vi "test-DiffDrvPoseEst2-testFollowTrajectory.vi"(0 "chassisSpeedsGenerator":refnum<vi>, 1 "TRAJECTORY":T10 {"States"."POSE"."ROTATION"."SIN" format="%13.4f"; "States"."POSE"."ROTATION"."COS" format="%13.4f"; "States"."POSE"."ROTATION"."VALUE" format="%13.4f"; "States"."POSE"."TRANSLATION"."Y" format="%14.3f"; "States"."POSE"."TRANSLATION"."X" format="%14.3f"; "TotalTImeSecs" format="%20.3f"}, 2 "DiffDrivePoseEstimate":T5 {"Diff_Drive_Odom_2"."M_PrevAngle"."SIN" format="%13.4f"; "Diff_Drive_Odom_2"."M_PrevAngle"."COS" format="%13.4f"; "Diff_Drive_Odom_2"."M_PrevAngle"."VALUE" format="%13.4f"; "Diff_Drive_Odom_2"."M_GyroOffset"."SIN" format="%13.4f"; "Diff_Drive_Odom_2"."M_GyroOffset"."COS" format="%13.4f"; "Diff_Drive_Odom_2"."M_GyroOffset"."VALUE" format="%13.4f"; "Diff_Drive_Odom_2"."M_POSE_Meters"."ROTATION"."SIN" format="%13.4f"; "Diff_Drive_Odom_2"."M_POSE_Meters"."ROTATION"."COS" format="%13.4f"; "Diff_Drive_Odom_2"."M_POSE_Meters"."ROTATION"."VALUE" format="%13.4f"; "Diff_Drive_Odom_2"."M_POSE_Meters"."TRANSLATION"."Y" format="%14.3f"; "Diff_Drive_Odom_2"."M_POSE_Meters"."TRANSLATION"."X" format="%14.3f"; "Diff_Drive_Kinematics"."TrackWidth_Meters" format="%20.4f"}, 3 "DIFF_DRIVE_KINEMATICS":T8 {"TrackWidth_Meters" format="%20.4f"}, 5 "genVisionMeasurement":refnum<vi>, 7 "StartingPose":T2={"TRANSLATION"={"X"=0.0, "Y"=0.0}, "ROTATION"={"VALUE"=0.0, "COS"=1.0, "SIN"=0.0}} {"ROTATION"."SIN" format="%13.4f"; "ROTATION"."COS" format="%13.4f"; "ROTATION"."VALUE" format="%13.4f"; "TRANSLATION"."Y" format="%14.3f"; "TRANSLATION"."X" format="%14.3f"}, 9 "EndingPose":T2={"TRANSLATION"={"X"=0.0, "Y"=0.0}, "ROTATION"={"VALUE"=0.0, "COS"=1.0, "SIN"=0.0}} {"ROTATION"."SIN" format="%13.4f"; "ROTATION"."COS" format="%13.4f"; "ROTATION"."VALUE" format="%13.4f"; "TRANSLATION"."Y" format="%14.3f"; "TRANSLATION"."X" format="%14.3f"}, 11 "dt_Seconds":dbl, 12 "VisionUpdateRate":dbl, 13 "VisionUpdateDelay":dbl, 14 "CheckError":bool) -> (4 "Test Passed":bool, 6 "Output Data":T1, 15 "DataForGraph":cluster{dbl[], dbl[]}[](array[cluster]))   [LabVIEW 2019]
uses:
  <vilib>/Rock Robotics/WPI/ThirdParty/JAS_Junk/TrajLib/TypeDef/TRAJECTORY.ctl
  <vilib>/Rock Robotics/WPI/ThirdParty/JAS_Junk/TrajLib/TypeDef/TRAJ_STATE.ctl
  <vilib>/Rock Robotics/WPI/ThirdParty/JAS_Junk/TrajLib/TypeDef/POSE2D.ctl
  <vilib>/Rock Robotics/WPI/ThirdParty/JAS_Junk/TrajLib/TypeDef/TRANSLATION2D.ctl
  <vilib>/Rock Robotics/WPI/ThirdParty/JAS_Junk/TrajLib/TypeDef/ROTATION2D.ctl
  <vilib>/Rock Robotics/WPI/ThirdParty/JAS_Junk/TrajLib/TypeDef/DIFF_DRIVE_KINEMATICS.ctl
  <vilib>/Rock Robotics/WPI/ThirdParty/JAS_Junk/TrajLib/TypeDef/DIFF_DRIVE_POSE_EST2.ctl
  <vilib>/Analysis/Matrix/Datatypes/RealMatrix.ctl
  <vilib>/Rock Robotics/WPI/ThirdParty/JAS_Junk/TrajLib/TypeDef/TIME_INTERPOLATABLE_VARIANT.ctl
  <vilib>/Rock Robotics/WPI/ThirdParty/JAS_Junk/TrajLib/TypeDef/DIFF_DRIVE_ODOM2.ctl
  <vilib>/Rock Robotics/WPI/ThirdParty/JAS_Junk/TrajLib/Conv_Deg_Radians.vi
  <vilib>/Rock Robotics/WPI/ThirdParty/JAS_Junk/TrajLib/VI/Util_GetTime_U32.vi
  <vilib>/Rock Robotics/WPI/ThirdParty/JAS_Junk/TrajLib/Pose2d_TransformBy.vi
  <vilib>/Rock Robotics/WPI/ThirdParty/JAS_Junk/TrajLib/VI/TimeInterpPose2d_CleanUp.vi
  <vilib>/Rock Robotics/WPI/ThirdParty/JAS_Junk/TrajLib/Rotation2d_RotateBy.vi
  <vilib>/Rock Robotics/WPI/ThirdParty/JAS_Junk/TrajLib/Rotation2d_UnaryMinus.vi
  <vilib>/Rock Robotics/WPI/ThirdParty/JAS_Junk/TrajLib/Util_CalcDist.vi
  <vilib>/Rock Robotics/WPI/ThirdParty/JAS_Junk/TrajLib/Translation2d_RotateBy.vi
  <vilib>/Rock Robotics/WPI/ThirdParty/JAS_Junk/TrajLib/Translation2d_Plus.vi
  <vilib>/Rock Robotics/WPI/ThirdParty/JAS_Junk/TrajLib/Pose2d_New_TRRO.vi
  <vilib>/Rock Robotics/WPI/ThirdParty/JAS_Junk/TrajLib/Rotation2d_CreateXY.vi
  <vilib>/Rock Robotics/WPI/ThirdParty/JAS_Junk/TrajLib/VI/Util_GetTime_U64.vi
  <vilib>/gmath/interp.llb/Search Ordered Table.vi
  <vilib>/Rock Robotics/WPI/ThirdParty/JAS_Junk/TrajLib/Trajectory_Library.lvlib
  <vilib>/Analysis/Matrix/NI_Matrix.lvlib
panel:
  in  "UseVIsion":bool=TRUE
  out "error out":errorcluster
  in  "error in (no error)":errorcluster
  # "<3, 1>"
  # "<3, 3>"
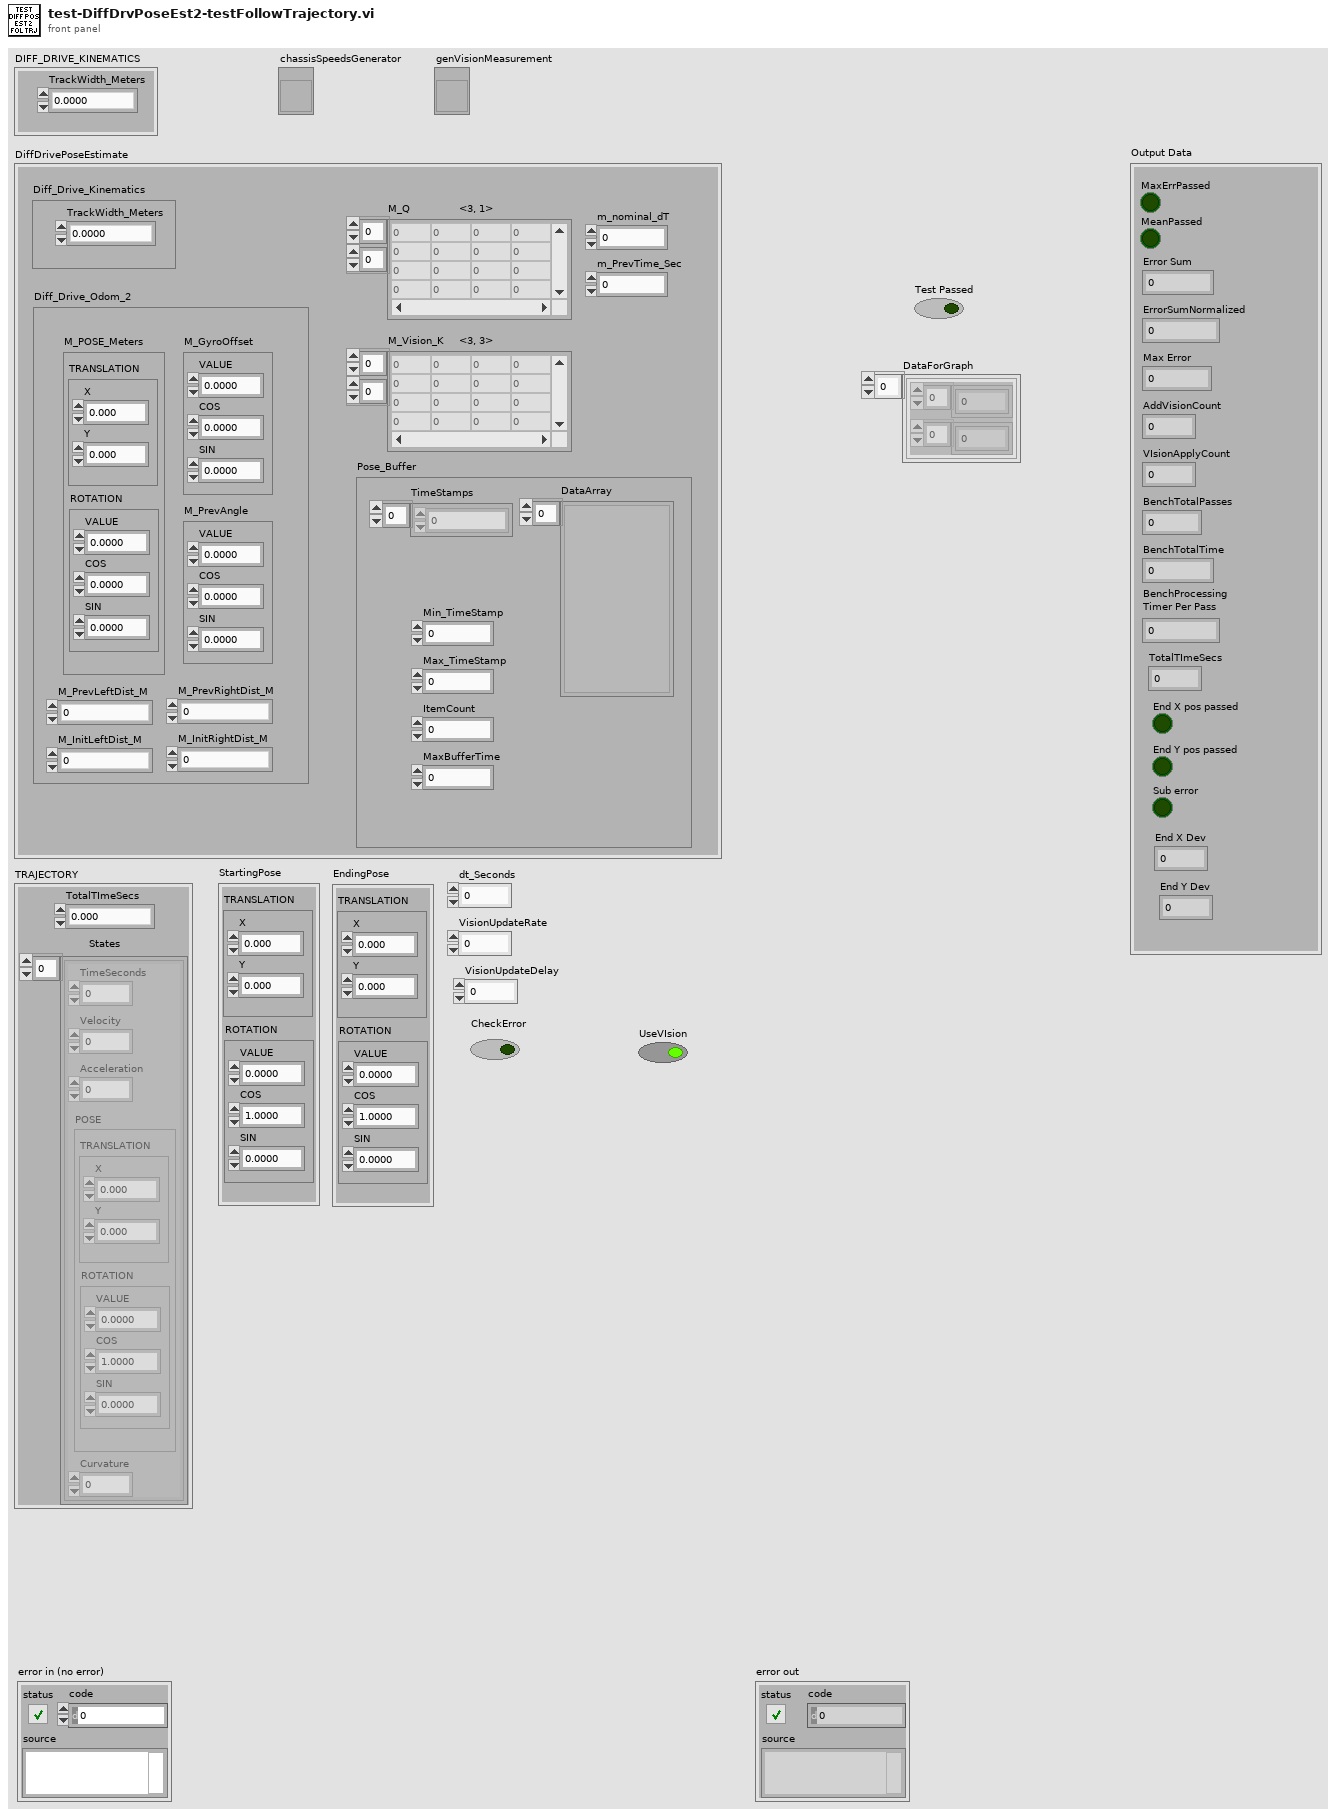
[diagram p1: front panel]
types:
  T1 = cluster{"MaxErrPassed":bool, "MeanPassed":bool, "Error Sum":dbl, "ErrorSumNormalized":dbl, "Max Error":dbl, "AddVisionCount":i32, "VIsionApplyCount":i32, "BenchTotalPasses":dbl, "BenchTotalTime":dbl, "BenchProcessing \nTimer Per Pass":dbl, "TotalTImeSecs":dbl, "End X pos passed":bool, "End Y pos passed":bool, "Sub error":bool, "End X Dev":dbl, "End Y Dev":dbl}
  T2 = typedef "Trajectory_Library.lvlib/POSE2D.ctl" = cluster{"TRANSLATION":T3, "ROTATION":T4}
  T3 = typedef "Trajectory_Library.lvlib/TRANSLATION2D.ctl" = cluster{"X":dbl, "Y":dbl}
  T4 = typedef "Trajectory_Library.lvlib/ROTATION2D.ctl" = cluster{"VALUE":dbl, "COS":dbl, "SIN":dbl}
  T5 = typedef "Trajectory_Library.lvlib/DIFF_DRIVE_POSE_EST2.ctl" = cluster{"M_Vision_K":T6, "m_nominal_dT":dbl, "m_PrevTime_Sec":dbl, "Pose_Buffer":T7, "Diff_Drive_Kinematics":T8, "Diff_Drive_Odom_2":T9, "M_Q":T6}
  T6 = typedef "NI_Matrix.lvlib/RealMatrix.ctl" = dbl[][]
  T7 = typedef "Trajectory_Library.lvlib/TIME_INTERPOLATABLE_VARIANT.ctl" = cluster{"TimeStamps":dbl[], "DataArray":variant[], "Min_TimeStamp":dbl, "Max_TimeStamp":dbl, "ItemCount":i32, "MaxBufferTime":dbl}
  T8 = typedef "Trajectory_Library.lvlib/DIFF_DRIVE_KINEMATICS.ctl" = cluster{"TrackWidth_Meters":dbl}
  T9 = typedef "Trajectory_Library.lvlib/DIFF_DRIVE_ODOM2.ctl" = cluster{"M_POSE_Meters":T2, "M_GyroOffset":T4, "M_PrevAngle":T4, "M_PrevLeftDist_M":dbl, "M_PrevRightDist_M":dbl, "M_InitLeftDist_M":dbl, "M_InitRightDist_M":dbl}
  T10 = typedef "Trajectory_Library.lvlib/TRAJECTORY.ctl" = cluster{"TotalTImeSecs":dbl, "States":T11[]}
  T11 = typedef "Trajectory_Library.lvlib/TRAJ_STATE.ctl" = cluster{"TimeSeconds":dbl, "Velocity":dbl, "Acceleration":dbl, "POSE":T2, "Curvature":dbl}
  T12 = typedef "Trajectory_Library.lvlib/TIME_INTERPOLATABLE_POSE2D.ctl" = cluster{"TimeStamps":dbl[], "Pose":T2[], "Min_TimeStamp":dbl, "Max_TimeStamp":dbl, "ItemCount":i32, "MaxBufferTime":dbl}
  T13 = typedef "Trajectory_Library.lvlib/TRANSFORM2D.ctl" = cluster{"TRANSLATION":T3, "ROTATION":T4, "xF":bool}
  T14 = typedef "Trajectory_Library.lvlib/CHASSIS_SPEEDS.ctl" = cluster{"vX":dbl, "vY":dbl, "vOmega":dbl}
  T15 = cluster{bool, bool, "Error Sum":dbl, dbl, dbl, i32, i32, "TotalPasses":dbl, "TotalTime":dbl, dbl, "TotalTImeSecs":dbl, bool, bool, bool, dbl, dbl}
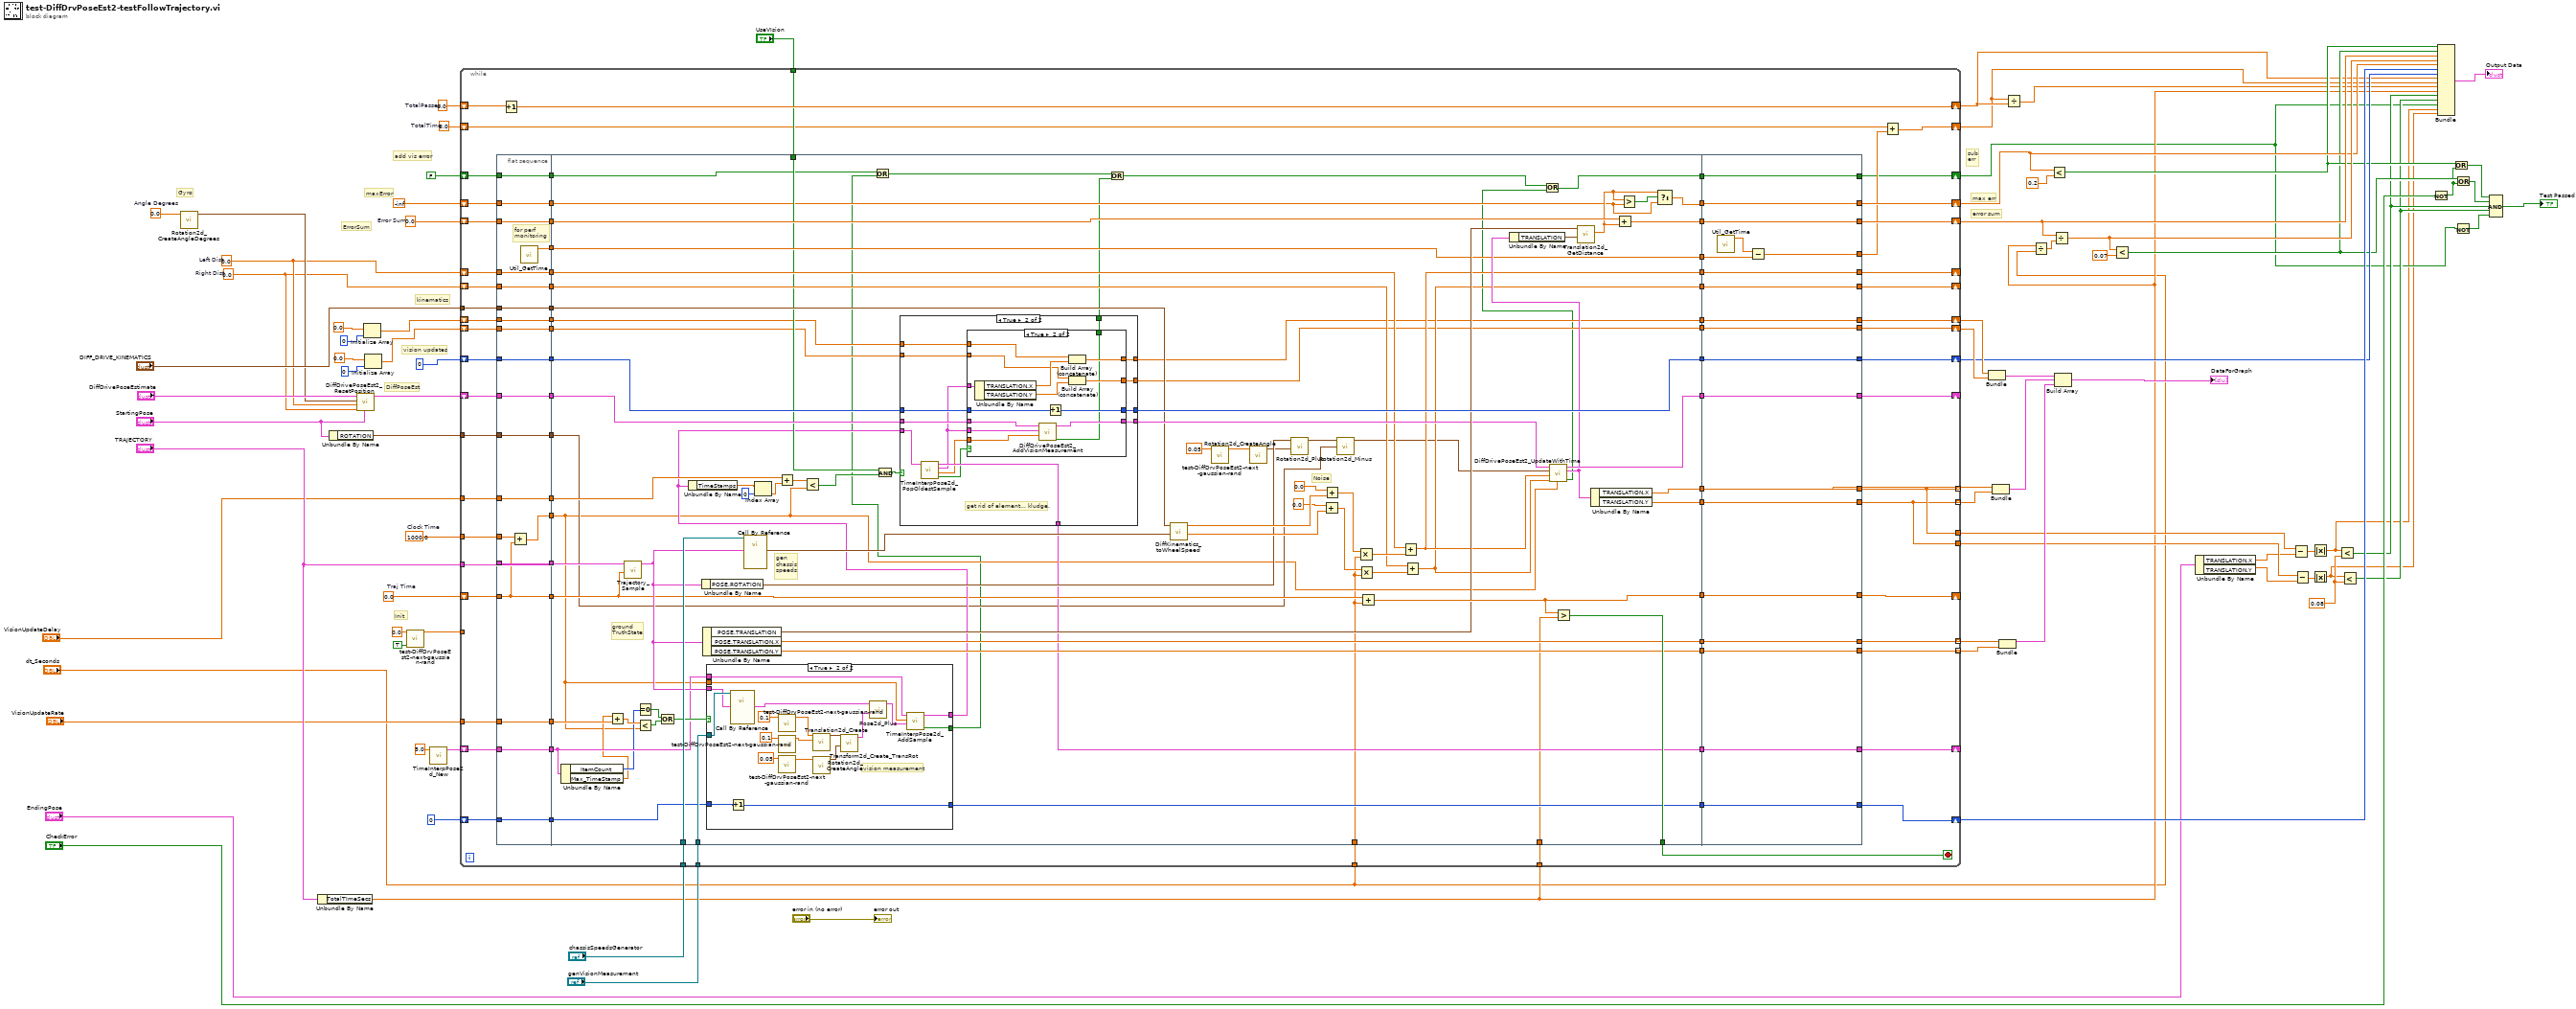
[diagram p0: block diagram]
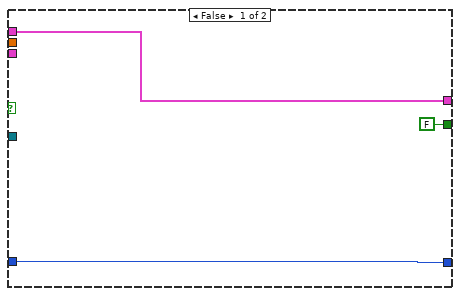
[diagram p2: hidden frame]
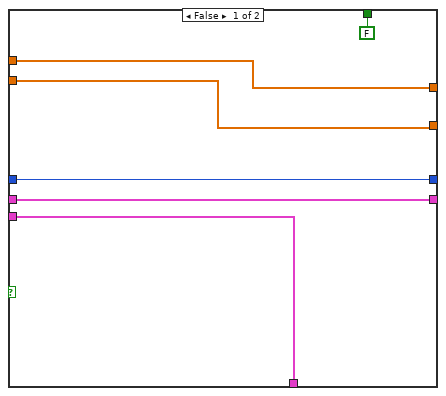
[diagram p3: hidden frame]
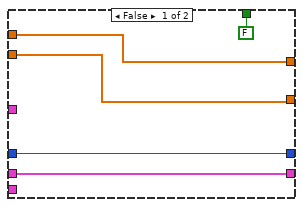
[diagram p4: hidden frame]
diagram:
  w22 = 0.08
  w47 = 1000.0  # Clock Time
  w57 = 0.0  # Angle Degrees
  w54 = 0.0  # Right Dist
  w55 = 0.0  # Left Dist
  w77 = 0.0  # TotalPasses
  w76 = 0.0  # TotalTime
  w71 = 0.0  # Error Sum
  w61 = 0.0  # Traj Time
  # "Init"
  # "sub\nerr"
  # "add vis error"
  # "max err"
  # "error sum"
  # "Gyro"
  # "ErrorSum"
  # "maxError"
  # "vision updates"
  # "kinematics"
  # "DiffPoseEst"
  n1 = call <vilib>:"Rotation2d_CreateAngleDegrees.vi"("Angle_Degrees"=w57) -> ("ROTATION"=w56:T4)  [unwired: 10 in]
  n2 = Unbundle By Name("TRAJECTORY") -> ("TotalTImeSecs"=w12:dbl)
  n3 = Unbundle By Name("StartingPose") -> ("ROTATION"=w30:T4)
  n4 = call <vilib>:"DiffDrivePoseEst2_ResetPosition.vi"("Pose"="StartingPose", "RightDistance_M"=w54, "LeftDistance_M"=w55, "Gyro"=w56, "in DiffDrivePoseEst2"="DiffDrivePoseEstimate") -> ("Out DiffDrivePoseEst2"=w58:T5)  [unwired: 6 in]
  n5 = Initialize Array(0.0, 0 ("dimension size")) -> (w42:dbl[])
  n6 = Initialize Array(0.0, 0 ("dimension size")) -> (w41:dbl[])
  n7 = call "test-DiffDrvPoseEst2-next-gaussian-rand.vi"("Init"=TRUE, "Multiplier"=0.0 ("R2")) -> ("Gaussian white noise"=w1:dbl)  [unwired: 9 in]
  n8 = call <vilib>:"TimeInterpPose2d_New.vi"("MaxTime"=5.0) -> ("TimeInterpPose"=w51:T12)  [unwired: 10 in]
  n9 = while {
    shift-right: [w162] -> _
    shift-left: w61 -> [w157]
    tunnel: "TRAJECTORY" -> [w160]
    tunnel: w12 -> [w161]
    tunnel: "VisionUpdateRate" -> [w110]
    shift-right: [w125] -> _
    shift-left: w58 -> [w159]
    tunnel: [w92] -> w62 mode=indexing
    tunnel: [w91] -> w63 mode=indexing
    shift-right: [w155] -> w32
    shift-left: 0 -> [w156]
    tunnel: [w154] -> w67 mode=indexing
    tunnel: [w153] -> w68 mode=indexing
    shift-right: [w150] -> w35
    shift-left: -inf -> [w149]
    shift-right: [w151] -> w37
    shift-left: w71 -> [w152]
    shift-right: [w87] -> w14
    shift-left: w76 -> [w88]
    shift-right: [w127] -> w15
    shift-left: w77 -> [w128]
    tunnel: "UseVIsion" -> [w126]
    shift-right: [w120] -> _
    shift-left: w55 -> [w123]
    shift-right: [w118] -> _
    shift-left: w54 -> [w121]
    tunnel: "DIFF_DRIVE_KINEMATICS" -> [w158]
    shift-right: [w113] -> _
    shift-left: w51 -> [w115]
    tunnel: "chassisSpeedsGenerator" -> [w116]
    tunnel: "genVisionMeasurement" -> [w111]
    tunnel: "VisionUpdateDelay" -> [w109]
    tunnel: w47 -> [w107]
    shift-right: [w102] -> w40
    shift-left: w42 -> [w105]
    shift-right: [w100] -> w39
    shift-left: w41 -> [w103]
    shift-right: [w96] -> w33
    shift-left: 0 -> [w97]
    tunnel: w30 -> [w93]
    tunnel: [w92] -> w28
    tunnel: [w91] -> w27
    shift-right: [w84] -> w7
    shift-left: FALSE -> [w85]
    tunnel: "dt_Seconds" -> [w82]
    tunnel: w1 -> [_]
    stop <- w148 stop-if-true
    n10 = flat-sequence {
      tunnel: w149 -> [w176]
      tunnel: w152 -> [w177]
      tunnel: w156 -> [w178]
      tunnel: w157 -> [w169]
      tunnel: w158 -> [w179]
      tunnel: w159 -> [w180]
      tunnel: w110 -> [w181]
      tunnel: w160 -> [w182]
      tunnel: [w182] -> w147
      tunnel: [w181] -> w146
      tunnel: [w180] -> w145
      tunnel: [w179] -> w144
      tunnel: [w169] -> w143
      tunnel: [w178] -> w142
      tunnel: [w177] -> w141
      tunnel: [w176] -> w140
      tunnel: [w171] -> w130
      tunnel: [w175] -> w124
      tunnel: w123 -> [w175]
      tunnel: [w174] -> w122
      tunnel: w121 -> [w174]
      tunnel: w115 -> [w173]
      tunnel: [w173] -> w114
      tunnel: w109 -> [w172]
      tunnel: [w172] -> w108
      tunnel: w107 -> [w170]
      tunnel: [w168] -> w106
      tunnel: w105 -> [w168]
      tunnel: [w167] -> w104
      tunnel: w103 -> [w167]
      tunnel: [w166] -> w98
      tunnel: w97 -> [w166]
      tunnel: [w165] -> w94
      tunnel: w93 -> [w165]
      tunnel: [w164] -> w90
      tunnel: [w163] -> w86
      tunnel: w85 -> [w163]
      tunnel: [w263] -> w148
      tunnel: w161 -> [w192]
      tunnel: w147 -> [w261]
      tunnel: w146 -> [w221]
      tunnel: w145 -> [w260]
      tunnel: w144 -> [w242]
      tunnel: w143 -> [w207]
      tunnel: w142 -> [w256]
      tunnel: w141 -> [w249]
      tunnel: w140 -> [w191]
      tunnel: [w262] -> w139
      tunnel: [w259] -> w138
      tunnel: [w258] -> w137
      tunnel: [w257] -> w136
      tunnel: [w255] -> w135
      tunnel: [w254] -> w134
      tunnel: [w253] -> w133
      tunnel: [w248] -> w132
      tunnel: [w245] -> w131
      tunnel: w130 -> [w244]
      tunnel: [w244] -> w129
      tunnel: w126 -> [w215]
      tunnel: w124 -> [w235]
      tunnel: w122 -> [w234]
      tunnel: [w231] -> w119
      tunnel: [w230] -> w117
      tunnel: w116 -> [w228]
      tunnel: w114 -> [w219]
      tunnel: [w206] -> w112
      tunnel: w111 -> [w226]
      tunnel: w108 -> [w212]
      tunnel: w106 -> [w205]
      tunnel: w104 -> [w204]
      tunnel: [w203] -> w101
      tunnel: [w202] -> w99
      tunnel: w98 -> [w201]
      tunnel: [w200] -> w95
      tunnel: w94 -> [w194]
      tunnel: w90 -> [w193]
      tunnel: w86 -> [w186]
      tunnel: [w188] -> w83
      tunnel: w82 -> [w183]
      tunnel: [w335] -> w150
      tunnel: [w336] -> w151
      tunnel: [w337] -> w153
      tunnel: [w338] -> w154
      tunnel: [w339] -> w155
      tunnel: [w340] -> w91
      tunnel: [w341] -> w92
      tunnel: [w342] -> w125
      tunnel: [w343] -> w162
      tunnel: w139 -> [w343]
      tunnel: w138 -> [w342]
      tunnel: w137 -> [w341]
      tunnel: w136 -> [w340]
      tunnel: w135 -> [w339]
      tunnel: w134 -> [w338]
      tunnel: w133 -> [w337]
      tunnel: w132 -> [w336]
      tunnel: w131 -> [w335]
      tunnel: w129 -> [w333]
      tunnel: [w332] -> w120
      tunnel: w119 -> [w332]
      tunnel: [w331] -> w118
      tunnel: w117 -> [w331]
      tunnel: [w330] -> w113
      tunnel: w112 -> [w330]
      tunnel: [w329] -> w102
      tunnel: w101 -> [w329]
      tunnel: [w328] -> w100
      tunnel: w99 -> [w328]
      tunnel: [w327] -> w96
      tunnel: w95 -> [w327]
      tunnel: [w326] -> w89
      tunnel: [w325] -> w84
      tunnel: w83 -> [w325]
      frame #0 {
        # "for perf\nmonitoring"
        n11 = Add(x=w170, y=w169) -> (x+y=w164:dbl)
        n12 = call <vilib>:"Util_GetTime.vi"() -> ("FPGA_Time_Seconds"=w171:dbl)  [unwired: 9 in, 2 out]
      }
      frame #1 {
        # "Noise"
        # "gen\nchassis\nspeeds"
        # "ground\nTruthState"
        n13 = Unbundle By Name(w219) -> ("ItemCount"=w218:i32, "Max_TimeStamp"=w217:dbl)
        n14 = Add(x=w217, y=w221) -> (x+y=w220:dbl)
        n15 = call <vilib>:"Trajectory_Sample.vi"("Time"=w207, "InputTRAJECTORY"=w261) -> ("OutputTRAJ_STATE"=w225:T11)  [unwired: 9 in]
        n16 = Equal To 0?(x=w218) -> (x = 0?=w224:bool)
        n17 = Less?(x=w220, y=w193) -> (x < y?=w223:bool)
        n18 = Compound Arithmetic op=OR(w224, w223) -> (w222:bool)
        n19 = Unbundle By Name(w225) -> ("POSE.ROTATION"=w233:T4)
        n20 = Unbundle By Name(w225) -> ("POSE.TRANSLATION"=w252:T3, "POSE.TRANSLATION.X"=w253:dbl, "POSE.TRANSLATION.Y"=w254:dbl)
        n21 = case shown="True" w222 {
          tunnel: w226 -> [_ w285]
          tunnel: w225 -> [_ w284]
          tunnel: w219 -> [w266 w273]
          tunnel: w193 -> [_ w271]
          tunnel: [w266 w270] -> w209
          tunnel: w201 -> [w265 w269]
          tunnel: [w265 w268] -> w200
          tunnel: [FALSE ("Error") w267] -> w184
          frame False {
          }
          frame True {
            # "vision measurement"
            n22 = Increment(x=w269) -> (x+1=w268:i32)
            n23 = call-by-ref "?"(reference=w285, "TRAJ_STATE"=w284) -> ("POSE2D"=w283:T2)  [unwired: 11 in, 2 out]
            n24 = call "test-DiffDrvPoseEst2-next-gaussian-rand.vi"("Multiplier"=0.1 ("R0")) -> ("Gaussian white noise"=w278:dbl)  [unwired: 10 in]
            n25 = call "test-DiffDrvPoseEst2-next-gaussian-rand.vi"("Multiplier"=0.1 ("R1")) -> ("Gaussian white noise"=w279:dbl)  [unwired: 10 in]
            n26 = call "test-DiffDrvPoseEst2-next-gaussian-rand.vi"("Multiplier"=0.05 ("R2")) -> ("Gaussian white noise"=w280:dbl)  [unwired: 10 in]
            n27 = call <vilib>:"Translation2d_Create.vi"("Y"=w279, "X"=w278) -> ("TRANSLATION"=w281:T3)  [unwired: 9 in]
            n28 = call <vilib>:"Rotation2d_CreateAngle.vi"("Angle"=w280) -> ("ROTATION"=w282:T4)  [unwired: 10 in]
            n29 = call <vilib>:"Transform2d_Create_TransRot.vi"("ROTATION"=w282, "TRANSLATION"=w281) -> ("TRANSFORM"=w274:T13)  [unwired: 9 in]
            n30 = call <vilib>:"Pose2d_Plus.vi"("other TRANSFORM"=w274, "in POSE"=w283) -> ("out POSE"=w272:T2)  [unwired: 9 in]
            n31 = call <vilib>:"TimeInterpPose2d_AddSample.vi"("Pose"=w272, "TimeStamp"=w271, "in TimeInterpPose"=w273) -> ("Error"=w267:bool, "out TimeInterpPose"=w270:T12)  [unwired: 7 in]
          }
        }
        n32 = Unbundle By Name(w209) -> ("TimeStamps"=w214:dbl[])
        n33 = call-by-ref "?"(reference=w228, "TRAJ_STATE"=w225) -> ("CHASSIS"=w227:T14)  [unwired: 11 in, 2 out]
        n34 = Index Array(array=w214, index=0) -> (element=w208:dbl)
        n35 = Add(x=w212, y=w208) -> (x+y=w211:dbl)
        n36 = Less?(x=w211, y=w193) -> (x < y?=w210:bool)
        n37 = Or(x=w186, y=w184) -> (x .or. y?=w185:bool)
        n38 = And(x=w215, y=w210) -> (x .and. y?=w216:bool)
        n39 = case shown="True" w216 {
          tunnel: w260 -> [w291 w305]
          tunnel: [w291 w304] -> w243
          tunnel: w256 -> [w290 w300]
          tunnel: [w290 w299] -> w255
          tunnel: w209 -> [w289 w303]
          tunnel: [w289 w302] -> w206
          tunnel: w205 -> [w288 w296]
          tunnel: w204 -> [w287 w295]
          tunnel: [w288 w294] -> w203
          tunnel: [w287 w293] -> w202
          tunnel: [FALSE ("Error") w292] -> w190
          frame False {
          }
          frame True {
            # "get rid of element... kludge."
            n40 = call <vilib>:"TimeInterpPose2d_PopOldestSample.vi"("in TimeInterpPose2d"=w303) -> ("Is Present"=w301:bool, "TimeStamp"=w298:dbl, "OutputPose2d"=w297:T2, "out TimeInterpPose2d"=w302:T12)  [unwired: 7 in]
            n41 = case shown="True" w301 {
              tunnel: w305 -> [w310 w324]
              tunnel: [w310 w323] -> w304
              tunnel: w300 -> [w309 w322]
              tunnel: [w309 w321] -> w299
              tunnel: w297 -> [_ w320]
              tunnel: w298 -> [_ w319]
              tunnel: w297 -> [_ w318]
              tunnel: w296 -> [w308 w315]
              tunnel: w295 -> [w307 w314]
              tunnel: [w308 w313] -> w294
              tunnel: [w307 w312] -> w293
              tunnel: [FALSE ("Error") w311] -> w292
              frame False {
              }
              frame True {
                n42 = Unbundle By Name(w318) -> ("TRANSLATION.X"=w317:dbl, "TRANSLATION.Y"=w316:dbl)
                n43 = call <vilib>:"DiffDrivePoseEst2_AddVisionMeasurement.vi"("TImeStamp_Seconds"=w319, "visionRobotPose"=w320, "in DiffDrivePoseEst2"=w324) -> ("Error"=w311:bool, "Out DiffDrivePoseEst2"=w323:T5)  [unwired: 7 in]
                n44 = Increment(x=w322) -> (x+1=w321:i32)
                n45 = Build Array (concatenate)(w315, w317) -> (w313:dbl[])
                n46 = Build Array (concatenate)(w314, w316) -> (w312:dbl[])
              }
            }
          }
        }
        n47 = Or(x=w185, y=w190) -> (x .or. y?=w189:bool)
        n48 = call <vilib>:"DiffKinematics_toWheelSpeed.vi"("CHASSIS Speed"=w227, "DIFF_DRIVE_KINEMATICS"=w242) -> ("RightVelocity"=w238:dbl, "LeftVelocity"=w241:dbl)  [unwired: 8 in]
        n49 = call "test-DiffDrvPoseEst2-next-gaussian-rand.vi"("Multiplier"=0.05 ("R0")) -> ("Gaussian white noise"=w229:dbl)  [unwired: 10 in]
        n50 = call <vilib>:"Rotation2d_CreateAngle.vi"("Angle"=w229) -> ("ROTATION"=w232:T4)  [unwired: 10 in]
        n51 = call <vilib>:"Rotation2d_Plus.vi"("other ROTATION"=w232, "in ROTATION"=w233) -> ("out ROTATION"=w197:T4)  [unwired: 9 in]
        n52 = Add(x=0.0, y=w238) -> (x+y=w240:dbl)
        n53 = Add(x=0.0, y=w241) -> (x+y=w239:dbl)
        n54 = call <vilib>:"Rotation2d_Minus.vi"("other ROTATION"=w194, "in ROTATION"=w197) -> ("out ROTATION"=w196:T4)  [unwired: 9 in]
        n55 = Multiply(x=w239, y=w183) -> (x*y=w236:dbl)
        n56 = Multiply(x=w240, y=w183) -> (x*y=w237:dbl)
        n57 = Add(x=w207, y=w183) -> (x+y=w262:dbl)
        n58 = Add(x=w235, y=w236) -> (x+y=w231:dbl)
        n59 = Add(x=w234, y=w237) -> (x+y=w230:dbl)
        n60 = call <vilib>:"DiffDrivePoseEst2_UpdateWithTime.vi"("CurrentTimeSeconds"=w193, "RightDistance"=w230, "LeftDistance"=w231, "GyroAngle"=w196, "in DiffDrivePoseEst2"=w243) -> ("Error"=w187:bool, "Estimated Pose"=w251:T2, "Out DiffDrivePoseEst2"=w259:T5)  [unwired: 4 in]
        n61 = Unbundle By Name(w251) -> ("TRANSLATION"=w250:T3)
        n62 = Or(x=w189, y=w187) -> (x .or. y?=w188:bool)
        n63 = Greater?(x=w262, y=w192) -> (0:w263:bool)
        n64 = call <vilib>:"Translation2d_GetDistance.vi"("other Translation"=w250, "In Translation"=w252) -> ("Distance"=w246:dbl)  [unwired: 9 in]
        n65 = Unbundle By Name(w251) -> ("TRANSLATION.X"=w258:dbl, "TRANSLATION.Y"=w257:dbl)
        n66 = Add(x=w249, y=w246) -> (x+y=w248:dbl)
        n67 = Greater?(x=w246, y=w191) -> (0:w247:bool)
        n68 = Select(t=w246, s=w247, f=w191) -> (s? t:f=w245:dbl)
      }
      frame #2 {
        n69 = call <vilib>:"Util_GetTime.vi"() -> ("FPGA_Time_Seconds"=w334:dbl)  [unwired: 9 in, 2 out]
        n70 = Subtract(x=w334, y=w333) -> (x-y=w326:dbl)
      }
    }
    n71 = Increment(x=w128) -> (x+1=w127:dbl)
    n72 = Add(x=w88, y=w89) -> (x+y=w87:dbl)
  }
  n73 = Bundle(w40, w39) -> (w64:cluster{dbl[], dbl[]})  [unwired: 1 in]
  n74 = Bundle(w62, w63) -> (w65:cluster{dbl[], dbl[]})  [unwired: 1 in]
  n75 = Bundle(w68, w67) -> (w69:cluster{dbl[], dbl[]})  [unwired: 1 in]
  n76 = Divide(x=w14, y=w15) -> (x/y=w13:dbl)
  n77 = Divide(x=w12, y="dt_Seconds") -> (x/y=w75:dbl)
  n78 = Less?(x=w35, y=0.2) -> (x < y?=w21:bool)
  n79 = Divide(x=w37, y=w75) -> (x/y=w36:dbl)
  n80 = Build Array(w64, w65, w69) -> (→"DataForGraph":cluster{dbl[], dbl[]}[])
  n81 = Less?(x=w36, y=0.07) -> (x < y?=w20:bool)
  n82 = Unbundle By Name("EndingPose") -> ("TRANSLATION.X"=w26:dbl, "TRANSLATION.Y"=w25:dbl)
  n83 = Subtract(x=w28, y=w26) -> (x-y=w24:dbl)
  n84 = Subtract(x=w27, y=w25) -> (x-y=w23:dbl)
  n85 = Absolute Value(x=w24) -> (abs(x)=w5:dbl)
  n86 = Absolute Value(x=w23) -> (abs(x)=w4:dbl)
  n87 = Less?(x=w5, y=w22) -> (x < y?=w11:bool)
  n88 = Less?(x=w4, y=w22) -> (x < y?=w10:bool)
  n89 = Not(x="CheckError") -> (.not. x?=w19:bool)
  n90 = Bundle(w21, w20, "Error Sum"=w37, w36, w35, w33, w32, "TotalPasses"=w15, "TotalTime"=w14, w13, "TotalTImeSecs"=w12, w11, w10, w7, w5, w4) -> (→"Output Data":T15)  [unwired: 1 in]
  n91 = Or(x=w21, y=w19) -> (x .or. y?=w17:bool)
  n92 = Or(x=w20, y=w19) -> (x .or. y?=w18:bool)
  n93 = Not(x=w7) -> (.not. x?=w8:bool)
  n94 = Compound Arithmetic op=AND(w17, w18, w11, w10, w8) -> (→"Test Passed":bool)
  "error out" <- "error in (no error)"
